vi "BigIntToString.vi"(1 "a":cluster{"Boolean":bool, "Array":u64[]}) -> (0 "String":string)   [LabVIEW 2023]
uses:
  <vilib>/Utility/error.llb/Trim Whitespace One-Sided.vi
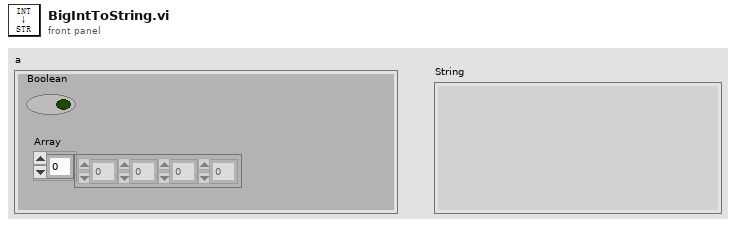
[diagram p1: front panel]
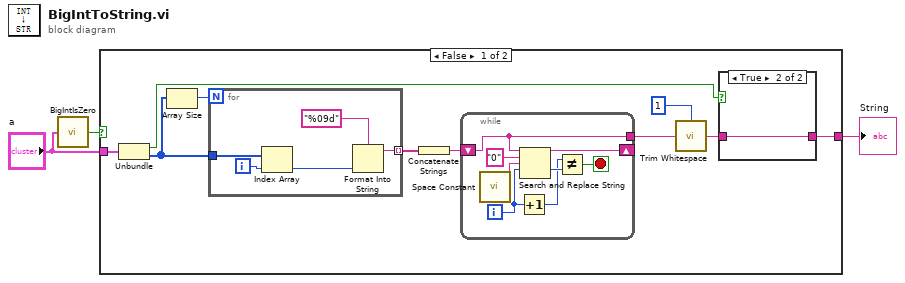
[diagram p0: block diagram]
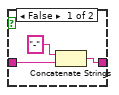
[diagram p2: hidden frame]
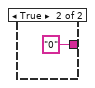
[diagram p3: hidden frame]
diagram:
  n1 = call "BigIntIsZero.vi"("a"="a") -> ("a = 0"=w2:bool)
  n2 = case shown="False" w2 {
    tunnel: "a" -> [w13 _]
    tunnel: [w8 "0"] -> w3
    frame False {
      n3 = Unbundle(w13) -> ("Boolean"=w9:bool, "Array"=w11:u64[])
      n4 = Array Size(array=w11) -> (size(s)=w12:i32)
      n5 = for {
        N: w12 -> [_]
        tunnel: w11 -> [w30]
        tunnel: [w26] -> w10 mode=indexing
        i -> [w29]
        n6 = Index Array(array=w30, index=w29) -> (element=w28:u64)
        n7 = Format Into String(format string="%09d", w28) -> (resulting string=w26:string)  [unwired: 2 in, 1 out]
      }
      n8 = Concatenate Strings(w10) -> (w7:string)
      n9 = while {
        shift-right: [w21] -> _
        shift-left: w7 -> [w16]
        tunnel: [w16] -> w4
        i -> [w15]
        stop <- w18 stop-if-true
        n10 = call <vilib>:"Space Constant.vi"() -> ("String"=w19:string)
        n11 = Increment(x=w15) -> (x+1=w14:i32)
        n12 = Search and Replace String(input string=w16, search string="0", replace string=w19, offset=w15) -> (result string=w21:string, offset past replacement=w17:i32)  [unwired: 4 in, 2 out]
        n13 = Not Equal?(x=w14, y=w17) -> (x != y?=w18:bool)
      }
      n14 = call <vilib>:"Trim Whitespace.vi"("string"=w4, "location (both)"=1) -> ("trimmed string"=w5:string)
      n15 = case shown="True" w9 {
        tunnel: w5 -> [w24 w25]
        tunnel: [w23 w25] -> w8
        frame False {
          n16 = Concatenate Strings("-", w24) -> (w23:string)
        }
        frame True {
        }
      }
    }
    frame True {
    }
  }
  "String" <- w3
